vi "Remove Item Reference from Tree.vi"(8 "error in":errorcluster, 11 "item ref":T1 format="%.0x") -> (0 "error out":errorcluster, 3 "removed":bool)   [LabVIEW 2020, in "Scan Engine Scripting.lvlib"]
uses:
  Scan Engine Scripting.lvlib
  <vilib>/NI VeriStand/Custom Device API/Custom Device Item Ref.ctl
  NationalInstruments.VeriStand.SystemDefinitionAPI
  <vilib>/NI VeriStand/Custom Device API/Custom Device API.lvlib
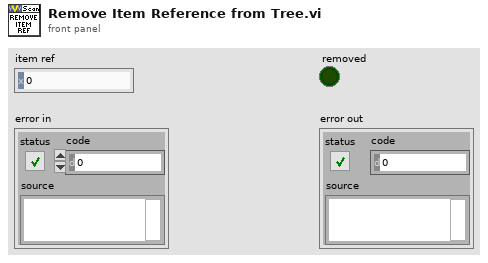
[diagram p1: front panel]
types:
  T1 = typedef "Custom Device API.lvlib/Custom Device Item Ref.ctl" = u64
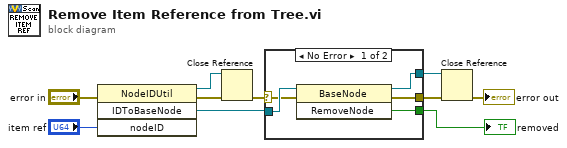
[diagram p0: block diagram]
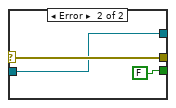
[diagram p2: hidden frame]
diagram:
  n1 = invoke class="NodeIDUtil" method="IDToBaseNode"(error in="error in", "nodeID"="item ref") -> (reference out=w9:refnum<k24>, error out=w8:errorcluster, "IDToBaseNode"=w5:refnum<k24>)  [unwired: 2 in, 1 out]
  n2 = Close Reference(reference=w9, error in (no error)=w8) -> (error out=w10:errorcluster)
  n3 = case shown="No Error" w10 {
    selector: w10 -> [w14 w18]
    tunnel: w5 -> [w15 w17]
    tunnel: [w13 w17] -> w2
    tunnel: [w12 w18] -> w3
    tunnel: [w11 FALSE ("RemoveNode")] -> w1
    frame No Error {
      n4 = invoke class="BaseNode" method="RemoveNode"(reference=w15, error in=w14) -> (reference out=w13:refnum<k24>, error out=w12:errorcluster, "RemoveNode"=w11:bool)  [unwired: 1 in]
    }
    frame Error {
    }
  }
  "removed" <- w1
  n5 = Close Reference(reference=w2, error in (no error)=w3) -> (error out=→"error out":errorcluster)
